vi "Set Package License.vi"(8 "error in (no error)":errorcluster, 10 "License":string, 11 "GitPackage in":refnum<class "GitPackage.lvclass">) -> (0 "error out":errorcluster, 3 "GitPackage out":refnum<class "GitPackage.lvclass">)   [LabVIEW 2020, in "GPack.lvlib" / "GitPackage.lvclass"]
uses:
  GitPackage.lvclass
  GitPackage.lvclass/GitPackage.ctl
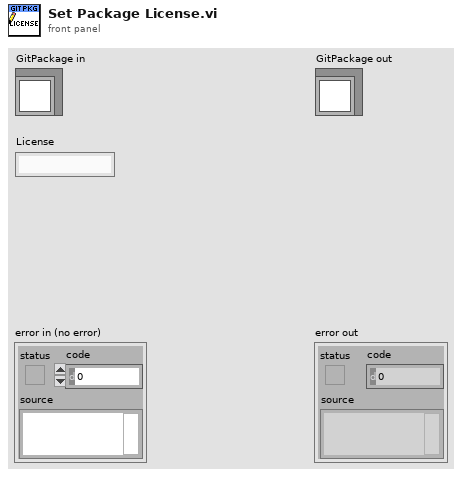
[diagram p1: front panel]
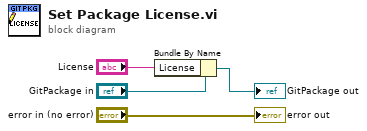
[diagram p0: block diagram]
diagram:
  n1 = Bundle By Name(cluster="GitPackage in", "License"="License") -> (→"GitPackage out":refnum<class "GitPackage.lvclass">)
  "error out" <- "error in (no error)"
